vi "Add Result Channels.vi"(8 "error in (no error)":errorcluster, 10 "Selected Waveform Tree items":T1[](array[typedef]) format="%.0x", 11 "WaveformCalculation in":refnum<class "WaveformCalculation.lvclass">) -> (0 "error out":errorcluster, 3 "WaveformCalculation out":refnum<class "WaveformCalculation.lvclass">)   [LabVIEW 2015, in "WaveformCalculation.lvclass"]
uses:
  WaveformCalculation.lvclass
  <vilib>/NI Veristand/Custom Device API/Custom Device Item Ref.ctl
  <vilib>/NI VeriStand/Custom Device API/Custom Device API.lvlib
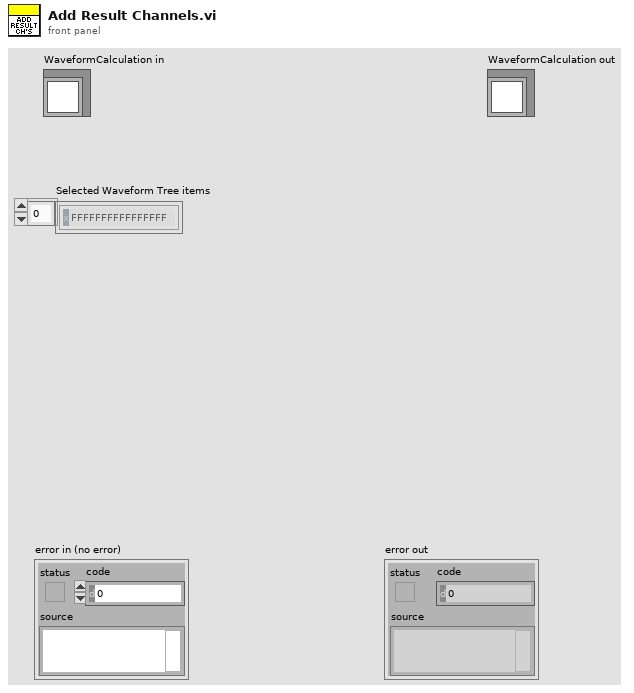
[diagram p1: front panel]
types:
  T1 = typedef "Custom Device API.lvlib/Custom Device Item Ref.ctl" = u64
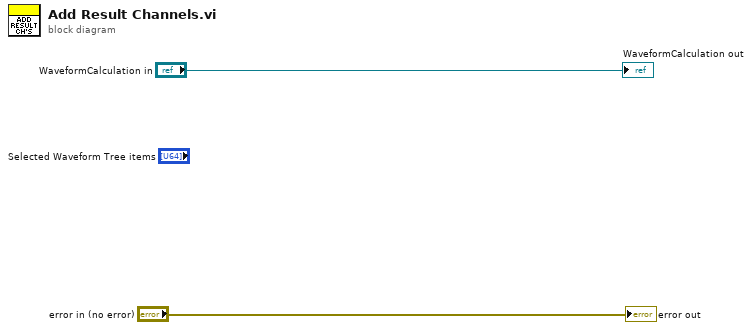
[diagram p0: block diagram]
diagram:
  "WaveformCalculation out" <- "WaveformCalculation in"
  "error out" <- "error in (no error)"
